vi "Configure Parametric Waveform.vi"(0 "VISA resource name":refnum<visa-resource-name>, 1 "Param. Wave Name":string, 2 "Prbs Parameters":cluster{"Prbs Type":u16, "Prbs Length [N]":i32}={"Prbs Type"=0, "Prbs Length [N]"=600} {"Prbs Type" items=[" PRBS-7", " PRBS-9", " PRBS-11", " PRBS-15", " PRBS-23", " PRBS-31"]}, 3 "Attribute":u16(ring) items=["Not Predefined", "Predefined"], 4 "Description":string, 5 "error in (no error)":errorcluster, 6 "Sampling Rate [Hz]":dbl=1200000000.0 format="%#_16g", 7 "Sine Parameters":T2={"Sine Cycles [N]"=1, "Sine Frequency [Hz]"=1000000.0, "Sine Phase [°]"=0, "Sine Length [N]"=600} {"Sine Frequency [Hz]" format="%#_16g"}, 8 "Sinc Parameters":T5={"Lobe Width [%]"=10.0, "Peak Position[%]"=50.0, "Sinc Length [N]"=600} {"Peak Position[%]" format="%#_16g"; "Lobe Width [%]" format="%#_16g"}, 9 "Exponential Parameters":T6={"Exponential Mode"=0, "Time Constant [s]"=5e-07, "Exp Length [N]"=600, "Exp Cycles [N]"=1} {"Time Constant [s]" format="%#_16g"; "Exponential Mode" items=["Rise", "Decay"]}, 10 "Auto Calc Option":u16(ring) items=["Length", "Sampling Rate", "Cycles", "Length & Cycles"], 11 "Pulse Parameters":T3={"Pulse Duty Cycle [%]"=50.0, "Pulse Pulse Delay[s]"=0.0, "Pulse Fall Time [s]"=1e-09, "Pulse Rise Time [s]"=1e-09, "Pulse Frequency [Hz]"=1000000.0, "Pulse Cycles [N]"=1, "Pulse Length [N]"=600} {"Pulse Frequency [Hz]" format="%#_16g"; "Pulse Rise Time [s]" format="%#_16g"; "Pulse Fall Time [s]" format="%#_16g"; "Pulse Pulse Delay[s]" format="%#_16g"; "Pulse Duty Cycle [%]" format="%#_16g"}, 12 "Wrap Around State":bool=TRUE, 13 "Sweep Parameters":T4={"Sweep Mode"=0, "Stop Frequency[Hz]"=5000000.0, "Start Frequency[Hz]"=1000000.0, "Sweep Length [N]"=600} {"Start Frequency[Hz]" format="%#_16g"; "Stop Frequency[Hz]" format="%#_16g"; "Sweep Mode" items=["Linear", "Logarithmic"]}, 15 "Square Parameters":T7={"Square Pulse Delay[s]"=0.0, "Sqaure Fall Time [s]"=1e-09, "Square Rise Time [s]"=1e-09, "Square Length [N]"=600, "Square Cycles [N]"=1, "Square Frequency [Hz]"=1000000.0} {"Square Frequency [Hz]" format="%#_16g"; "Square Rise Time [s]" format="%#_16g"; "Sqaure Fall Time [s]" format="%#_16g"; "Square Pulse Delay[s]" format="%#_16e"}, 16 "Multitone Parameters":T8(array[cluster])=[{"Tone Amplitude  [V]"=1.0, "Tone Phase  [°]"=0.0, "Tone Frequency [Hz]"=1000000.0}] {"Tone Frequency [Hz]" format="%#_16g"; "Tone Phase  [°]" format="%#_16g"; "Tone Amplitude  [V]" format="%#_16g"}, 18 "Parametric Type":u16(ring) items=["Sine", "Pulse", "Sweep", "Sinc", "Exponential", "Prbs", "Square", "Multitone"]) -> (14 "VISA resource name out":refnum<visa-resource-name>, 19 "error out":errorcluster)   [LabVIEW 2020, in "Active Technologies AWG3000.lvlib"]
uses:
  Active Technologies AWG3000.lvlib
panel:
  in  "Parametric Type Tabs":T1(tab)
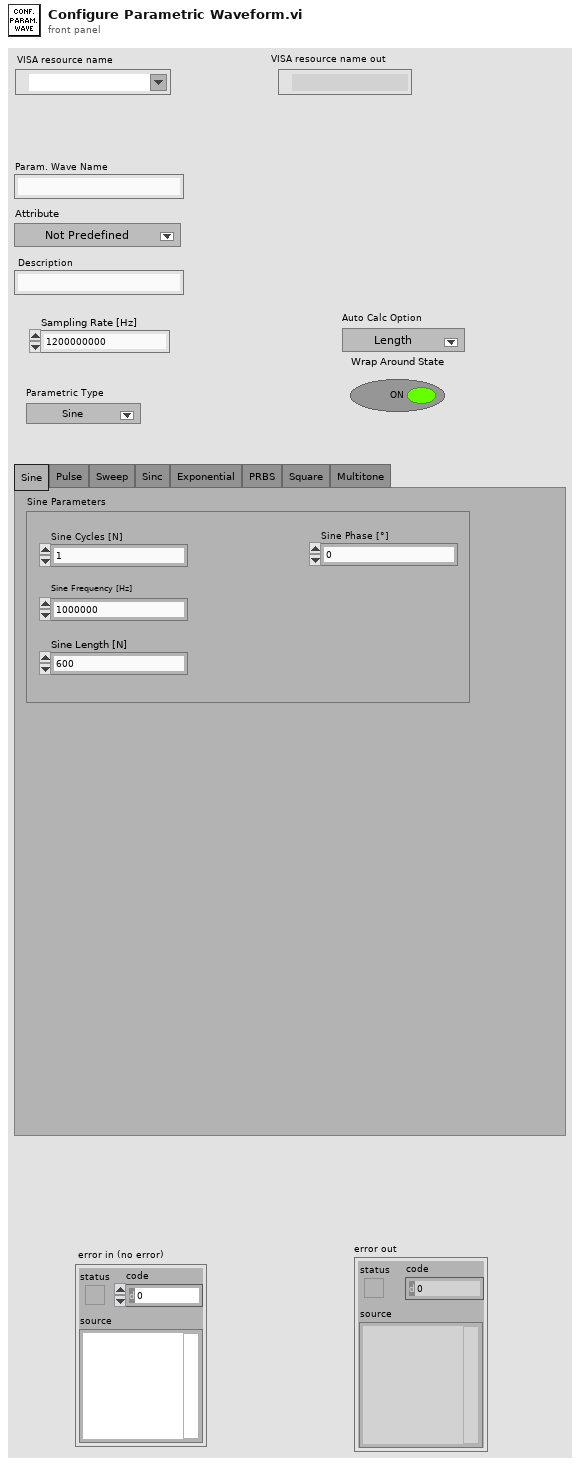
[diagram p1: front panel]
types:
  T1 = enum32{"Sine", "Pulse", "Sweep", "Sinc", "Exponential", "PRBS", "Square", "Multitone"}
  T2 = cluster{"Sine Cycles [N]":u32, "Sine Frequency [Hz]":dbl, "Sine Phase [°]":u32, "Sine Length [N]":i32}
  T3 = cluster{"Pulse Duty Cycle [%]":dbl, "Pulse Pulse Delay[s]":dbl, "Pulse Fall Time [s]":dbl, "Pulse Rise Time [s]":dbl, "Pulse Frequency [Hz]":dbl, "Pulse Cycles [N]":u32, "Pulse Length [N]":i32}
  T4 = cluster{"Sweep Mode":u16, "Stop Frequency[Hz]":dbl, "Start Frequency[Hz]":dbl, "Sweep Length [N]":i32}
  T5 = cluster{"Lobe Width [%]":dbl, "Peak Position[%]":dbl, "Sinc Length [N]":i32}
  T6 = cluster{"Exponential Mode":u16, "Time Constant [s]":dbl, "Exp Length [N]":i32, "Exp Cycles [N]":u32}
  T7 = cluster{"Square Pulse Delay[s]":dbl, "Sqaure Fall Time [s]":dbl, "Square Rise Time [s]":dbl, "Square Length [N]":i32, "Square Cycles [N]":u32, "Square Frequency [Hz]":dbl}
  T8 = cluster{"Tone Amplitude  [V]":dbl, "Tone Phase  [°]":dbl, "Tone Frequency [Hz]":dbl}[]
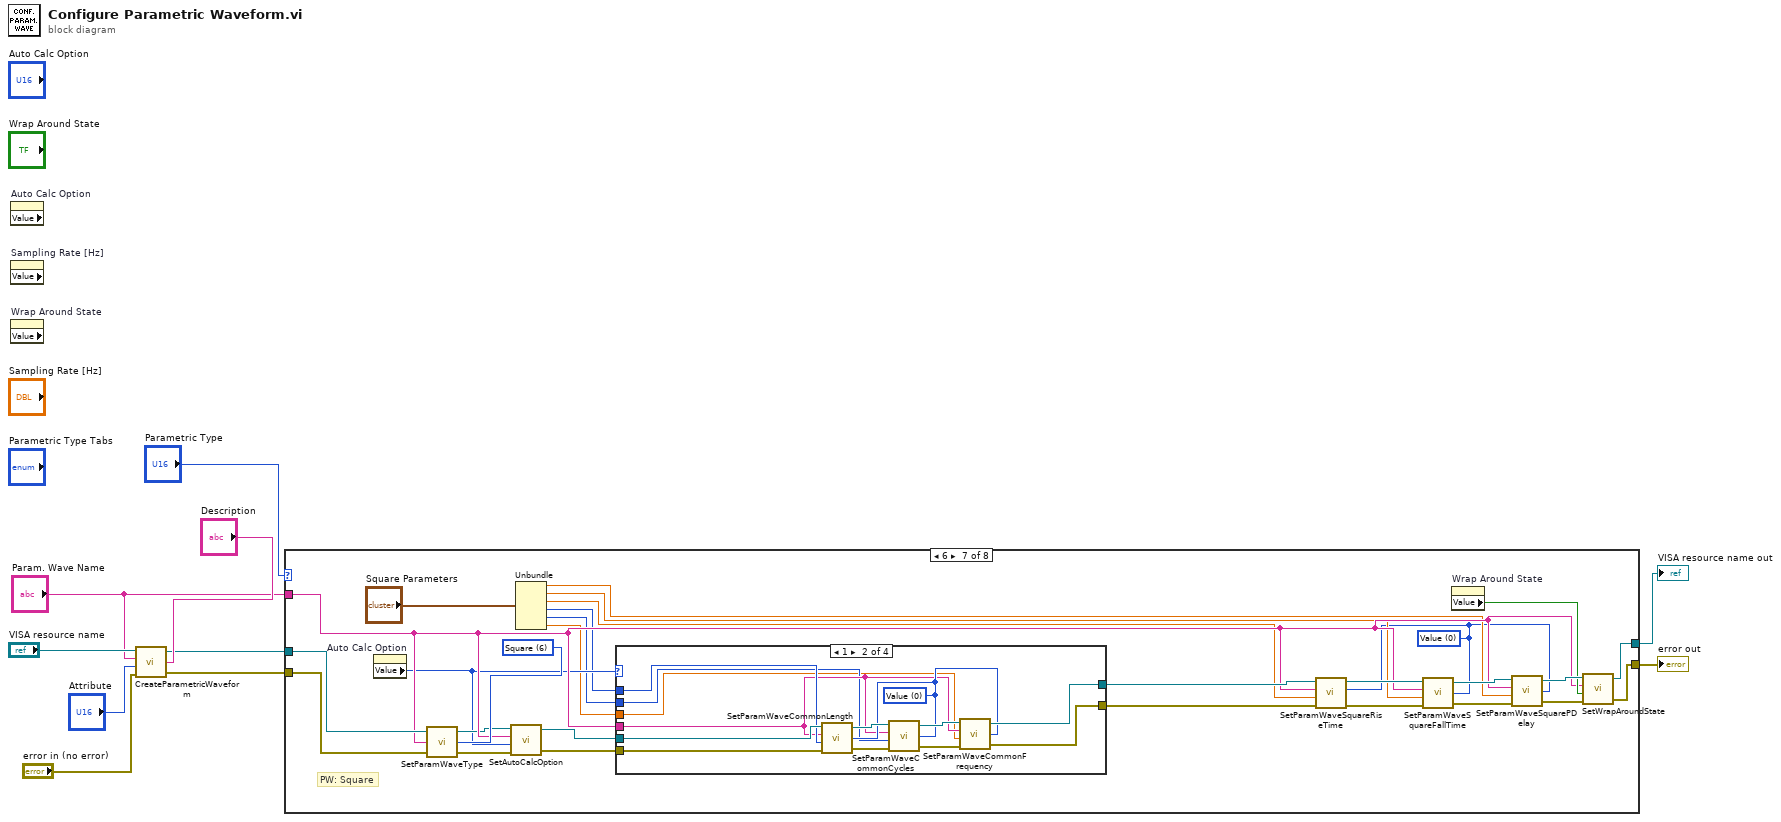
[diagram p0: block diagram]
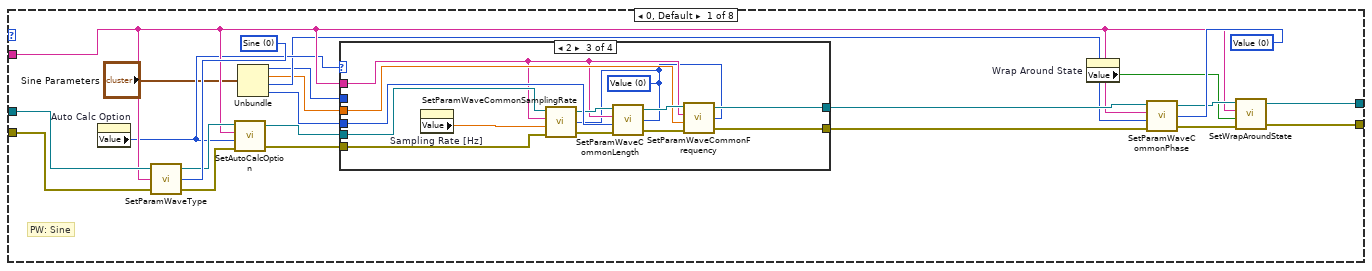
[diagram p2: hidden frame]
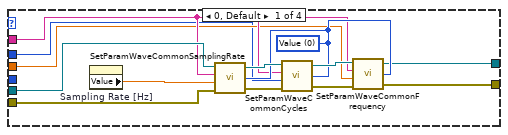
[diagram p3: hidden frame]
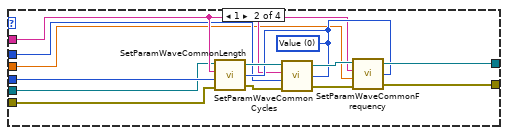
[diagram p4: hidden frame]
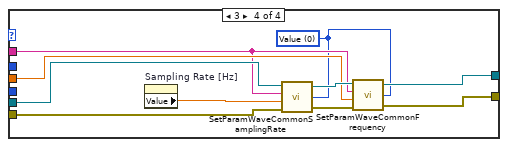
[diagram p5: hidden frame]
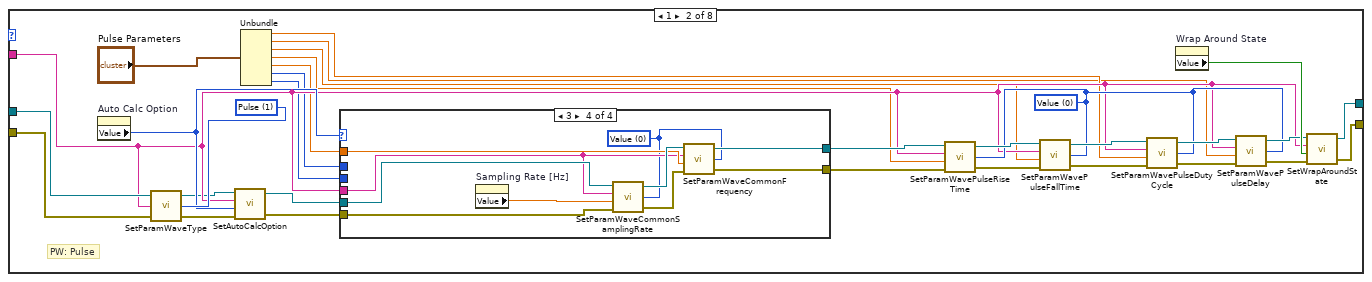
[diagram p6: hidden frame]
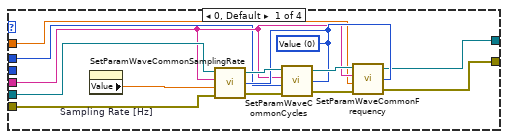
[diagram p7: hidden frame]
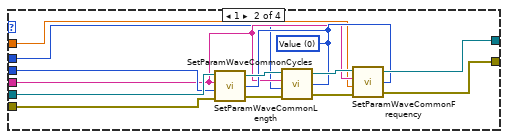
[diagram p8: hidden frame]
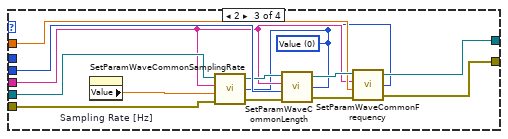
[diagram p9: hidden frame]
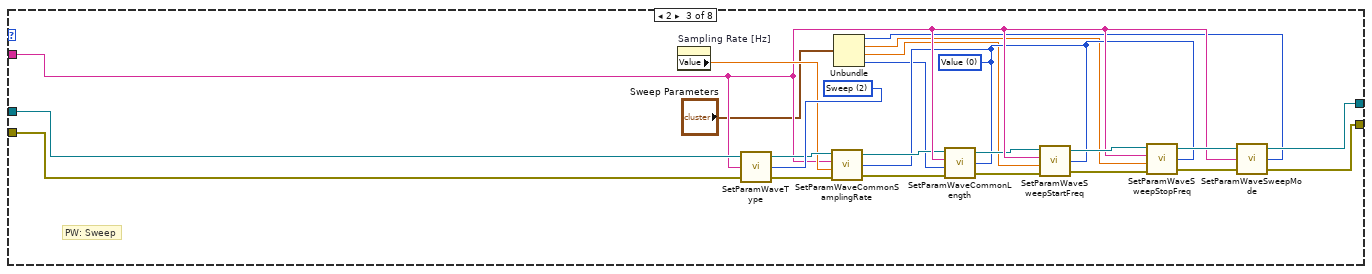
[diagram p10: hidden frame]
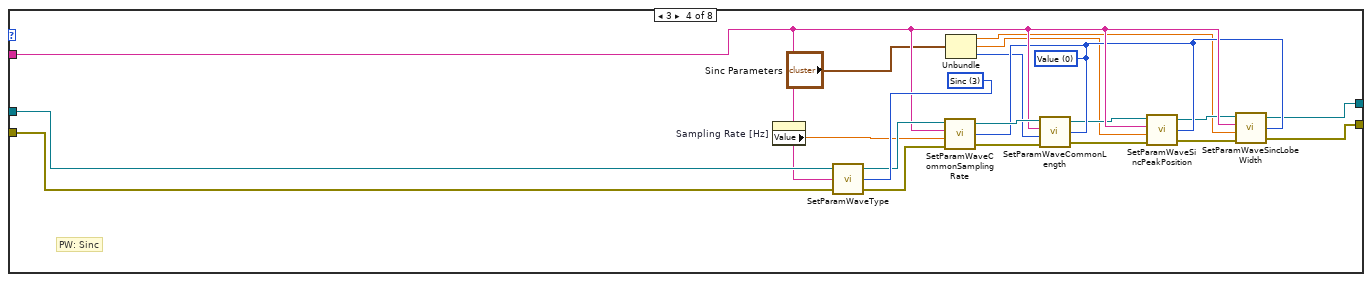
[diagram p11: hidden frame]
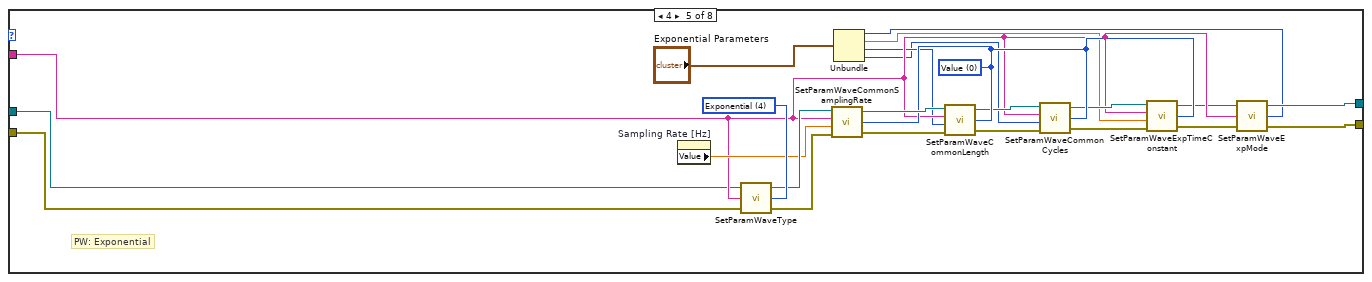
[diagram p12: hidden frame]
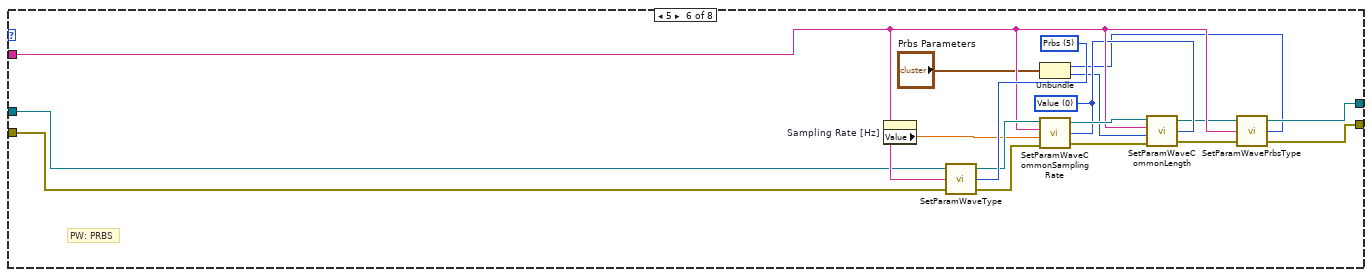
[diagram p13: hidden frame]
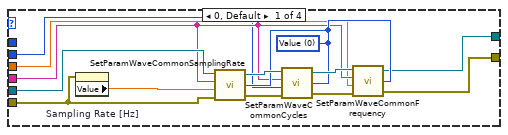
[diagram p14: hidden frame]
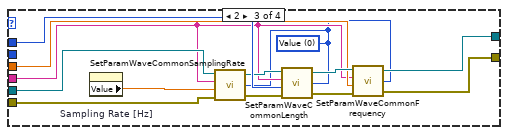
[diagram p15: hidden frame]
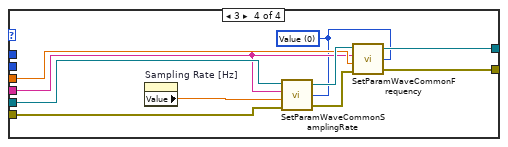
[diagram p16: hidden frame]
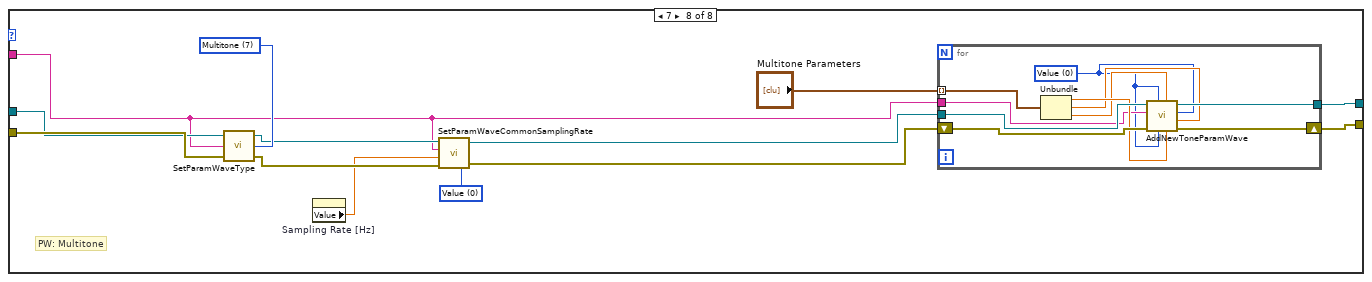
[diagram p17: hidden frame]
diagram:
  n1 = property on="Auto Calc Option" class="Ring (strict)" props=["Value"]() -> ()  [unwired: 2 in, 3 out]
  n2 = property on="Sampling Rate [Hz]" class="DigNum (strict)" props=["Value"]() -> ()  [unwired: 2 in, 3 out]
  n3 = property on="Wrap Around State" class="Bool (strict)" props=["Value"]() -> ()  [unwired: 2 in, 3 out]
  n4 = call "CreateParametricWaveform.vi"("Description"="Description", "error in (no error)"="error in (no error)", "Attribute"="Attribute", "Param. Wave Name"="Param. Wave Name", "VISA resource name"="VISA resource name") -> ("error out"=w4:errorcluster, "VISA resource name out"=w5:refnum<visa-resource-name>)
  n5 = case shown="6" "Parametric Type" {
    tunnel: "Param. Wave Name" -> [w19 w94 w172 w196 w217 w238 w258 w322]
    tunnel: w5 -> [w32 w110 w183 w198 w210 w237 w271 w333]
    tunnel: w4 -> [w31 w109 w182 w197 w211 w236 w270 w334]
    tunnel: [w23 w105 w181 w190 w213 w232 w266 w330] -> w2
    tunnel: [w22 w106 w180 w189 w212 w231 w265 w329] -> w3
    frame 0, Default {
      w27 = u16 0 items=["Value", "Default", "Minimum", "Maximum"] ("Selection")
      w30 = u16 0 items=["Sine", "Pulse", "Sweep", "Sinc", "Exponential", "Prbs", "Square", "Multitone"] ("ParamWaveType")
      # "PW: Sine"
      n6 = property on="Auto Calc Option" class="Ring (strict)"() -> ("Value"=w18:u16)  [unwired: 2 in, 2 out]
      n7 = call "SetParamWaveType.vi"("ParamWaveType"=w30, "error in (no error)"=w31, "ParamWave Name"=w19, "VISA resource name"=w32) -> ("error out"=w21:errorcluster, "VISA resource name out"=w20:refnum<visa-resource-name>)
      n8 = call "SetAutoCalcOption.vi"("error in (no error)"=w21, "Auto Calc Option"=w18, "ParamWave Name"=w19, "VISA resource name"=w20) -> ("error out"=w17:errorcluster, "VISA resource name out"=w16:refnum<visa-resource-name>)  [unwired: 1 in]
      n9 = Unbundle("Sine Parameters") -> ("Sine Cycles [N]"=w11:u32, "Sine Frequency [Hz]"=w13:dbl, "Sine Phase [°]"=w14:u32, "Sine Length [N]"=w12:i32)
      n10 = case shown="2" w18 {
        tunnel: w16 -> [w44 w46 w70 w81]
        tunnel: w17 -> [w43 w58 w69 w79]
        tunnel: w19 -> [w35 w50 w60 w75]
        tunnel: [w37 w52 w61 w73] -> w29
        tunnel: [w36 w53 w62 w74] -> w28
        tunnel: w13 -> [w34 w47 w63 w76]
        tunnel: w11 -> [w33 w49 _ _]
        tunnel: w12 -> [_ w57 w68 _]
        frame 0, Default {
          w38 = u16 0 items=["Value", "Default", "Minimum", "Maximum"] ("Selection")
          n11 = property on="Sampling Rate [Hz]" class="DigNum (strict)"() -> ("Value"=w45:dbl)  [unwired: 2 in, 2 out]
          n12 = call "SetParamWaveCommonSamplingRate.vi"("Selection"=w38, "error in (no error)"=w43, "Sampling Rate [Hz]"=w45, "ParamWave Name"=w35, "VISA resource name"=w44) -> ("error out"=w42:errorcluster, "VISA resource name out"=w41:refnum<visa-resource-name>)
          n13 = call "SetParamWaveCommonCycles.vi"("Selection"=w38, "error in (no error)"=w42, "Cycles [N]"=w33, "ParamWave Name"=w35, "VISA resource name"=w41) -> ("error out"=w39:errorcluster, "VISA resource name out"=w40:refnum<visa-resource-name>)
          n14 = call "SetParamWaveCommonFrequency.vi"("Selection"=w38, "error in (no error)"=w39, "Frequency [Hz]"=w34, "ParamWave Name"=w35, "VISA resource name"=w40) -> ("error out"=w37:errorcluster, "VISA resource name out"=w36:refnum<visa-resource-name>)
        }
        frame 1 {
          w51 = u16 0 items=["Value", "Default", "Minimum", "Maximum"] ("Selection")
          n15 = call "SetParamWaveCommonLength.vi"("Selection"=w51, "error in (no error)"=w58, "Length [N]"=w57, "ParamWave Name"=w50, "VISA resource name"=w46) -> ("error out"=w55:errorcluster, "VISA resource name out"=w56:refnum<visa-resource-name>)
          n16 = call "SetParamWaveCommonCycles.vi"("Selection"=w51, "error in (no error)"=w55, "Cycles [N]"=w49, "ParamWave Name"=w50, "VISA resource name"=w56) -> ("error out"=w48:errorcluster, "VISA resource name out"=w54:refnum<visa-resource-name>)
          n17 = call "SetParamWaveCommonFrequency.vi"("Selection"=w51, "error in (no error)"=w48, "Frequency [Hz]"=w47, "ParamWave Name"=w50, "VISA resource name"=w54) -> ("error out"=w52:errorcluster, "VISA resource name out"=w53:refnum<visa-resource-name>)
        }
        frame 2 {
          w59 = u16 0 items=["Value", "Default", "Minimum", "Maximum"] ("Selection")
          n18 = property on="Sampling Rate [Hz]" class="DigNum (strict)"() -> ("Value"=w71:dbl)  [unwired: 2 in, 2 out]
          n19 = call "SetParamWaveCommonSamplingRate.vi"("Selection"=w59, "error in (no error)"=w69, "Sampling Rate [Hz]"=w71, "ParamWave Name"=w60, "VISA resource name"=w70) -> ("error out"=w66:errorcluster, "VISA resource name out"=w67:refnum<visa-resource-name>)
          n20 = call "SetParamWaveCommonLength.vi"("Selection"=w59, "error in (no error)"=w66, "Length [N]"=w68, "ParamWave Name"=w60, "VISA resource name"=w67) -> ("error out"=w64:errorcluster, "VISA resource name out"=w65:refnum<visa-resource-name>)
          n21 = call "SetParamWaveCommonFrequency.vi"("Selection"=w59, "error in (no error)"=w64, "Frequency [Hz]"=w63, "ParamWave Name"=w60, "VISA resource name"=w65) -> ("error out"=w61:errorcluster, "VISA resource name out"=w62:refnum<visa-resource-name>)
        }
        frame 3 {
          w72 = u16 0 items=["Value", "Default", "Minimum", "Maximum"] ("Selection")
          n22 = property on="Sampling Rate [Hz]" class="DigNum (strict)"() -> ("Value"=w80:dbl)  [unwired: 2 in, 2 out]
          n23 = call "SetParamWaveCommonSamplingRate.vi"("Selection"=w72, "error in (no error)"=w79, "Sampling Rate [Hz]"=w80, "ParamWave Name"=w75, "VISA resource name"=w81) -> ("error out"=w77:errorcluster, "VISA resource name out"=w78:refnum<visa-resource-name>)
          n24 = call "SetParamWaveCommonFrequency.vi"("Selection"=w72, "error in (no error)"=w77, "Frequency [Hz]"=w76, "ParamWave Name"=w75, "VISA resource name"=w78) -> ("error out"=w73:errorcluster, "VISA resource name out"=w74:refnum<visa-resource-name>)
        }
      }
      n25 = property on="Wrap Around State" class="Bool (strict)"() -> ("Value"=w24:bool)  [unwired: 2 in, 2 out]
      n26 = call "SetParamWaveCommonPhase.vi"("Selection"=w27, "error in (no error)"=w29, "Phase [°]"=w14, "ParamWave Name"=w19, "VISA resource name"=w28) -> ("error out"=w25:errorcluster, "VISA resource name out"=w26:refnum<visa-resource-name>)
      n27 = call "SetWrapAroundState.vi"("error in (no error)"=w25, "Wrap Around State"=w24, "ParamWave Name"=w19, "VISA resource name"=w26) -> ("error out"=w22:errorcluster, "VISA resource name out"=w23:refnum<visa-resource-name>)  [unwired: 1 in]
    }
    frame 1 {
      w96 = u16 0 items=["Value", "Default", "Minimum", "Maximum"] ("Selection")
      w112 = u16 1 items=["Sine", "Pulse", "Sweep", "Sinc", "Exponential", "Prbs", "Square", "Multitone"] ("ParamWaveType")
      # "PW: Pulse"
      n28 = property on="Auto Calc Option" class="Ring (strict)"() -> ("Value"=w95:u16)  [unwired: 2 in, 2 out]
      n29 = call "SetParamWaveType.vi"("ParamWaveType"=w112, "error in (no error)"=w109, "ParamWave Name"=w94, "VISA resource name"=w110) -> ("error out"=w93:errorcluster, "VISA resource name out"=w92:refnum<visa-resource-name>)
      n30 = call "SetAutoCalcOption.vi"("error in (no error)"=w93, "Auto Calc Option"=w95, "ParamWave Name"=w94, "VISA resource name"=w92) -> ("error out"=w91:errorcluster, "VISA resource name out"=w90:refnum<visa-resource-name>)  [unwired: 1 in]
      n31 = Unbundle("Pulse Parameters") -> ("Pulse Duty Cycle [%]"=w88:dbl, "Pulse Pulse Delay[s]"=w87:dbl, "Pulse Fall Time [s]"=w86:dbl, "Pulse Rise Time [s]"=w85:dbl, "Pulse Frequency [Hz]"=w84:dbl, "Pulse Cycles [N]"=w83:u32, "Pulse Length [N]"=w82:i32)
      n32 = case shown="3" w95 {
        tunnel: w90 -> [w124 w138 w150 w161]
        tunnel: w91 -> [w123 w137 w149 w159]
        tunnel: w94 -> [w115 w129 w140 w155]
        tunnel: [w117 w131 w141 w153] -> w103
        tunnel: [w116 w132 w142 w154] -> w104
        tunnel: w84 -> [w114 w126 w143 w156]
        tunnel: w83 -> [w113 w128 _ _]
        tunnel: w82 -> [_ w136 w148 _]
        frame 0, Default {
          w118 = u16 0 items=["Value", "Default", "Minimum", "Maximum"] ("Selection")
          n33 = property on="Sampling Rate [Hz]" class="DigNum (strict)"() -> ("Value"=w125:dbl)  [unwired: 2 in, 2 out]
          n34 = call "SetParamWaveCommonSamplingRate.vi"("Selection"=w118, "error in (no error)"=w123, "Sampling Rate [Hz]"=w125, "ParamWave Name"=w115, "VISA resource name"=w124) -> ("error out"=w122:errorcluster, "VISA resource name out"=w121:refnum<visa-resource-name>)
          n35 = call "SetParamWaveCommonCycles.vi"("Selection"=w118, "error in (no error)"=w122, "Cycles [N]"=w113, "ParamWave Name"=w115, "VISA resource name"=w121) -> ("error out"=w119:errorcluster, "VISA resource name out"=w120:refnum<visa-resource-name>)
          n36 = call "SetParamWaveCommonFrequency.vi"("Selection"=w118, "error in (no error)"=w119, "Frequency [Hz]"=w114, "ParamWave Name"=w115, "VISA resource name"=w120) -> ("error out"=w117:errorcluster, "VISA resource name out"=w116:refnum<visa-resource-name>)
        }
        frame 1 {
          w130 = u16 0 items=["Value", "Default", "Minimum", "Maximum"] ("Selection")
          n37 = call "SetParamWaveCommonLength.vi"("Selection"=w130, "error in (no error)"=w137, "Length [N]"=w136, "ParamWave Name"=w129, "VISA resource name"=w138) -> ("error out"=w134:errorcluster, "VISA resource name out"=w135:refnum<visa-resource-name>)
          n38 = call "SetParamWaveCommonCycles.vi"("Selection"=w130, "error in (no error)"=w134, "Cycles [N]"=w128, "ParamWave Name"=w129, "VISA resource name"=w135) -> ("error out"=w127:errorcluster, "VISA resource name out"=w133:refnum<visa-resource-name>)
          n39 = call "SetParamWaveCommonFrequency.vi"("Selection"=w130, "error in (no error)"=w127, "Frequency [Hz]"=w126, "ParamWave Name"=w129, "VISA resource name"=w133) -> ("error out"=w131:errorcluster, "VISA resource name out"=w132:refnum<visa-resource-name>)
        }
        frame 2 {
          w139 = u16 0 items=["Value", "Default", "Minimum", "Maximum"] ("Selection")
          n40 = property on="Sampling Rate [Hz]" class="DigNum (strict)"() -> ("Value"=w151:dbl)  [unwired: 2 in, 2 out]
          n41 = call "SetParamWaveCommonSamplingRate.vi"("Selection"=w139, "error in (no error)"=w149, "Sampling Rate [Hz]"=w151, "ParamWave Name"=w140, "VISA resource name"=w150) -> ("error out"=w146:errorcluster, "VISA resource name out"=w147:refnum<visa-resource-name>)
          n42 = call "SetParamWaveCommonLength.vi"("Selection"=w139, "error in (no error)"=w146, "Length [N]"=w148, "ParamWave Name"=w140, "VISA resource name"=w147) -> ("error out"=w144:errorcluster, "VISA resource name out"=w145:refnum<visa-resource-name>)
          n43 = call "SetParamWaveCommonFrequency.vi"("Selection"=w139, "error in (no error)"=w144, "Frequency [Hz]"=w143, "ParamWave Name"=w140, "VISA resource name"=w145) -> ("error out"=w141:errorcluster, "VISA resource name out"=w142:refnum<visa-resource-name>)
        }
        frame 3 {
          w152 = u16 0 items=["Value", "Default", "Minimum", "Maximum"] ("Selection")
          n44 = property on="Sampling Rate [Hz]" class="DigNum (strict)"() -> ("Value"=w160:dbl)  [unwired: 2 in, 2 out]
          n45 = call "SetParamWaveCommonSamplingRate.vi"("Selection"=w152, "error in (no error)"=w159, "Sampling Rate [Hz]"=w160, "ParamWave Name"=w155, "VISA resource name"=w161) -> ("error out"=w157:errorcluster, "VISA resource name out"=w158:refnum<visa-resource-name>)
          n46 = call "SetParamWaveCommonFrequency.vi"("Selection"=w152, "error in (no error)"=w157, "Frequency [Hz]"=w156, "ParamWave Name"=w155, "VISA resource name"=w158) -> ("error out"=w153:errorcluster, "VISA resource name out"=w154:refnum<visa-resource-name>)
        }
      }
      n47 = call "SetParamWavePulseRiseTime.vi"("Selection"=w96, "error in (no error)"=w103, "Rise Time [s]"=w85, "ParamWave Name"=w94, "VISA resource name"=w104) -> ("error out"=w102:errorcluster, "VISA resource name out"=w101:refnum<visa-resource-name>)
      n48 = call "SetParamWavePulseFallTime.vi"("Selection"=w96, "error in (no error)"=w102, "Fall Time [s]"=w86, "ParamWave Name"=w94, "VISA resource name"=w101) -> ("error out"=w97:errorcluster, "VISA resource name out"=w100:refnum<visa-resource-name>)
      n49 = call "SetParamWavePulseDutyCycle.vi"("Selection"=w96, "error in (no error)"=w97, "Duty Cycle [%]"=w88, "ParamWave Name"=w94, "VISA resource name"=w100) -> ("error out"=w98:errorcluster, "VISA resource name out"=w99:refnum<visa-resource-name>)
      n50 = property on="Wrap Around State" class="Bool (strict)"() -> ("Value"=w111:bool)  [unwired: 2 in, 2 out]
      n51 = call "SetParamWavePulseDelay.vi"("Selection"=w96, "error in (no error)"=w98, "Pulse Delay[s]"=w87, "ParamWave Name"=w94, "VISA resource name"=w99) -> ("error out"=w107:errorcluster, "VISA resource name out"=w108:refnum<visa-resource-name>)
      n52 = call "SetWrapAroundState.vi"("error in (no error)"=w107, "Wrap Around State"=w111, "ParamWave Name"=w94, "VISA resource name"=w108) -> ("error out"=w106:errorcluster, "VISA resource name out"=w105:refnum<visa-resource-name>)  [unwired: 1 in]
    }
    frame 2 {
      w167 = u16 0 items=["Value", "Default", "Minimum", "Maximum"] ("Selection")
      w184 = u16 2 items=["Sine", "Pulse", "Sweep", "Sinc", "Exponential", "Prbs", "Square", "Multitone"] ("ParamWaveType")
      # "PW: Sweep"
      n53 = property on="Sampling Rate [Hz]" class="DigNum (strict)"() -> ("Value"=w175:dbl)  [unwired: 2 in, 2 out]
      n54 = call "SetParamWaveType.vi"("ParamWaveType"=w184, "error in (no error)"=w182, "ParamWave Name"=w172, "VISA resource name"=w183) -> ("error out"=w177:errorcluster, "VISA resource name out"=w176:refnum<visa-resource-name>)
      n55 = call "SetParamWaveCommonSamplingRate.vi"("Selection"=w167, "error in (no error)"=w177, "Sampling Rate [Hz]"=w175, "ParamWave Name"=w172, "VISA resource name"=w176) -> ("error out"=w170:errorcluster, "VISA resource name out"=w171:refnum<visa-resource-name>)
      n56 = Unbundle("Sweep Parameters") -> ("Sweep Mode"=w165:u16, "Stop Frequency[Hz]"=w164:dbl, "Start Frequency[Hz]"=w162:dbl, "Sweep Length [N]"=w163:i32)
      n57 = call "SetParamWaveCommonLength.vi"("Selection"=w167, "error in (no error)"=w170, "Length [N]"=w163, "ParamWave Name"=w172, "VISA resource name"=w171) -> ("error out"=w168:errorcluster, "VISA resource name out"=w169:refnum<visa-resource-name>)
      n58 = call "SetParamWaveSweepStartFreq.vi"("Selection"=w167, "error in (no error)"=w168, "Start Frequency[Hz]"=w162, "ParamWave Name"=w172, "VISA resource name"=w169) -> ("error out"=w178:errorcluster, "VISA resource name out"=w174:refnum<visa-resource-name>)
      n59 = call "SetParamWaveSweepStopFreq.vi"("Selection"=w167, "error in (no error)"=w178, "Stop Frequency[Hz]"=w164, "ParamWave Name"=w172, "VISA resource name"=w174) -> ("error out"=w179:errorcluster, "VISA resource name out"=w173:refnum<visa-resource-name>)
      n60 = call "SetParamWaveSweepMode.vi"("Sweep Mode"=w165, "error in (no error)"=w179, "ParamWave Name"=w172, "VISA resource name"=w173) -> ("error out"=w180:errorcluster, "VISA resource name out"=w181:refnum<visa-resource-name>)
    }
    frame 3 {
      w195 = u16 0 items=["Value", "Default", "Minimum", "Maximum"] ("Selection")
      w204 = u16 3 items=["Sine", "Pulse", "Sweep", "Sinc", "Exponential", "Prbs", "Square", "Multitone"] ("ParamWaveType")
      # "PW: Sinc"
      n61 = property on="Sampling Rate [Hz]" class="DigNum (strict)"() -> ("Value"=w201:dbl)  [unwired: 2 in, 2 out]
      n62 = call "SetParamWaveType.vi"("ParamWaveType"=w204, "error in (no error)"=w197, "ParamWave Name"=w196, "VISA resource name"=w198) -> ("error out"=w203:errorcluster, "VISA resource name out"=w202:refnum<visa-resource-name>)
      n63 = call "SetParamWaveCommonSamplingRate.vi"("Selection"=w195, "error in (no error)"=w203, "Sampling Rate [Hz]"=w201, "ParamWave Name"=w196, "VISA resource name"=w202) -> ("error out"=w199:errorcluster, "VISA resource name out"=w200:refnum<visa-resource-name>)
      n64 = Unbundle("Sinc Parameters") -> ("Lobe Width [%]"=w187:dbl, "Peak Position[%]"=w186:dbl, "Sinc Length [N]"=w185:i32)
      n65 = call "SetParamWaveCommonLength.vi"("Selection"=w195, "error in (no error)"=w199, "Length [N]"=w185, "ParamWave Name"=w196, "VISA resource name"=w200) -> ("error out"=w193:errorcluster, "VISA resource name out"=w194:refnum<visa-resource-name>)
      n66 = call "SetParamWaveSincPeakPosition.vi"("Selection"=w195, "error in (no error)"=w193, "Peak Position[%]"=w186, "ParamWave Name"=w196, "VISA resource name"=w194) -> ("error out"=w191:errorcluster, "VISA resource name out"=w192:refnum<visa-resource-name>)
      n67 = call "SetParamWaveSincLobeWidth.vi"("Selection"=w195, "error in (no error)"=w191, "Lobe Width [%]"=w187, "ParamWave Name"=w196, "VISA resource name"=w192) -> ("error out"=w189:errorcluster, "VISA resource name out"=w190:refnum<visa-resource-name>)
    }
    frame 4 {
      w221 = u16 0 items=["Value", "Default", "Minimum", "Maximum"] ("Selection")
      w227 = u16 4 items=["Sine", "Pulse", "Sweep", "Sinc", "Exponential", "Prbs", "Square", "Multitone"] ("ParamWaveType")
      # "PW: Exponential"
      n68 = property on="Sampling Rate [Hz]" class="DigNum (strict)"() -> ("Value"=w224:dbl)  [unwired: 2 in, 2 out]
      n69 = call "SetParamWaveType.vi"("ParamWaveType"=w227, "error in (no error)"=w211, "ParamWave Name"=w217, "VISA resource name"=w210) -> ("error out"=w226:errorcluster, "VISA resource name out"=w225:refnum<visa-resource-name>)
      n70 = call "SetParamWaveCommonSamplingRate.vi"("Selection"=w221, "error in (no error)"=w226, "Sampling Rate [Hz]"=w224, "ParamWave Name"=w217, "VISA resource name"=w225) -> ("error out"=w222:errorcluster, "VISA resource name out"=w223:refnum<visa-resource-name>)
      n71 = Unbundle("Exponential Parameters") -> ("Exponential Mode"=w208:u16, "Time Constant [s]"=w207:dbl, "Exp Length [N]"=w206:i32, "Exp Cycles [N]"=w205:u32)
      n72 = call "SetParamWaveCommonLength.vi"("Selection"=w221, "error in (no error)"=w222, "Length [N]"=w206, "ParamWave Name"=w217, "VISA resource name"=w223) -> ("error out"=w219:errorcluster, "VISA resource name out"=w220:refnum<visa-resource-name>)
      n73 = call "SetParamWaveCommonCycles.vi"("Selection"=w221, "error in (no error)"=w219, "Cycles [N]"=w205, "ParamWave Name"=w217, "VISA resource name"=w220) -> ("error out"=w216:errorcluster, "VISA resource name out"=w218:refnum<visa-resource-name>)
      n74 = call "SetParamWaveExpTimeConstant.vi"("Selection"=w221, "error in (no error)"=w216, "Time Constant [s]"=w207, "ParamWave Name"=w217, "VISA resource name"=w218) -> ("error out"=w214:errorcluster, "VISA resource name out"=w215:refnum<visa-resource-name>)
      n75 = call "SetParamWaveExpMode.vi"("Exponential Mode"=w208, "error in (no error)"=w214, "ParamWave Name"=w217, "VISA resource name"=w215) -> ("error out"=w212:errorcluster, "VISA resource name out"=w213:refnum<visa-resource-name>)
    }
    frame 5 {
      w235 = u16 0 items=["Value", "Default", "Minimum", "Maximum"] ("Selection")
      w244 = u16 5 items=["Sine", "Pulse", "Sweep", "Sinc", "Exponential", "Prbs", "Square", "Multitone"] ("ParamWaveType")
      # "PW: PRBS"
      n76 = property on="Sampling Rate [Hz]" class="DigNum (strict)"() -> ("Value"=w241:dbl)  [unwired: 2 in, 2 out]
      n77 = call "SetParamWaveType.vi"("ParamWaveType"=w244, "error in (no error)"=w236, "ParamWave Name"=w238, "VISA resource name"=w237) -> ("error out"=w243:errorcluster, "VISA resource name out"=w242:refnum<visa-resource-name>)
      n78 = Unbundle("Prbs Parameters") -> ("Prbs Type"=w229:u16, "Prbs Length [N]"=w228:i32)
      n79 = call "SetParamWaveCommonSamplingRate.vi"("Selection"=w235, "error in (no error)"=w243, "Sampling Rate [Hz]"=w241, "ParamWave Name"=w238, "VISA resource name"=w242) -> ("error out"=w239:errorcluster, "VISA resource name out"=w240:refnum<visa-resource-name>)
      n80 = call "SetParamWaveCommonLength.vi"("Selection"=w235, "error in (no error)"=w239, "Length [N]"=w228, "ParamWave Name"=w238, "VISA resource name"=w240) -> ("error out"=w233:errorcluster, "VISA resource name out"=w234:refnum<visa-resource-name>)
      n81 = call "SetParamWavePrbsType.vi"("Prbs Type"=w229, "error in (no error)"=w233, "ParamWave Name"=w238, "VISA resource name"=w234) -> ("error out"=w231:errorcluster, "VISA resource name out"=w232:refnum<visa-resource-name>)
    }
    frame 6 {
      w245 = u16 0 items=["Value", "Default", "Minimum", "Maximum"] ("Selection")
      w272 = u16 6 items=["Sine", "Pulse", "Sweep", "Sinc", "Exponential", "Prbs", "Square", "Multitone"] ("ParamWaveType")
      # "PW: Square"
      n82 = property on="Auto Calc Option" class="Ring (strict)"() -> ("Value"=w253:u16)  [unwired: 2 in, 2 out]
      n83 = call "SetParamWaveType.vi"("ParamWaveType"=w272, "error in (no error)"=w270, "ParamWave Name"=w258, "VISA resource name"=w271) -> ("error out"=w256:errorcluster, "VISA resource name out"=w257:refnum<visa-resource-name>)
      n84 = call "SetAutoCalcOption.vi"("error in (no error)"=w256, "Auto Calc Option"=w253, "ParamWave Name"=w258, "VISA resource name"=w257) -> ("error out"=w254:errorcluster, "VISA resource name out"=w255:refnum<visa-resource-name>)  [unwired: 1 in]
      n85 = Unbundle("Square Parameters") -> ("Square Pulse Delay[s]"=w246:dbl, "Sqaure Fall Time [s]"=w251:dbl, "Square Rise Time [s]"=w250:dbl, "Square Length [N]"=w247:i32, "Square Cycles [N]"=w248:u32, "Square Frequency [Hz]"=w249:dbl)
      n86 = case shown="1" w253 {
        tunnel: w255 -> [w285 w298 w311 w321]
        tunnel: w254 -> [w274 w297 w310 w320]
        tunnel: w258 -> [w277 w289 w301 w316]
        tunnel: [w279 w291 w302 w314] -> w263
        tunnel: [w278 w292 w303 w315] -> w264
        tunnel: w249 -> [w276 w286 w304 w317]
        tunnel: w248 -> [w275 w288 _ _]
        tunnel: w247 -> [_ w296 w309 _]
        frame 0, Default {
          w280 = u16 0 items=["Value", "Default", "Minimum", "Maximum"] ("Selection")
          n87 = property on="Sampling Rate [Hz]" class="DigNum (strict)"(error in=w274) -> ("Value"=w273:dbl)  [unwired: 1 in, 2 out]
          n88 = call "SetParamWaveCommonSamplingRate.vi"("Selection"=w280, "error in (no error)"=w274, "Sampling Rate [Hz]"=w273, "ParamWave Name"=w277, "VISA resource name"=w285) -> ("error out"=w284:errorcluster, "VISA resource name out"=w283:refnum<visa-resource-name>)
          n89 = call "SetParamWaveCommonCycles.vi"("Selection"=w280, "error in (no error)"=w284, "Cycles [N]"=w275, "ParamWave Name"=w277, "VISA resource name"=w283) -> ("error out"=w281:errorcluster, "VISA resource name out"=w282:refnum<visa-resource-name>)
          n90 = call "SetParamWaveCommonFrequency.vi"("Selection"=w280, "error in (no error)"=w281, "Frequency [Hz]"=w276, "ParamWave Name"=w277, "VISA resource name"=w282) -> ("error out"=w279:errorcluster, "VISA resource name out"=w278:refnum<visa-resource-name>)
        }
        frame 1 {
          w290 = u16 0 items=["Value", "Default", "Minimum", "Maximum"] ("Selection")
          n91 = call "SetParamWaveCommonLength.vi"("Selection"=w290, "error in (no error)"=w297, "Length [N]"=w296, "ParamWave Name"=w289, "VISA resource name"=w298) -> ("error out"=w294:errorcluster, "VISA resource name out"=w295:refnum<visa-resource-name>)
          n92 = call "SetParamWaveCommonCycles.vi"("Selection"=w290, "error in (no error)"=w294, "Cycles [N]"=w288, "ParamWave Name"=w289, "VISA resource name"=w295) -> ("error out"=w287:errorcluster, "VISA resource name out"=w293:refnum<visa-resource-name>)
          n93 = call "SetParamWaveCommonFrequency.vi"("Selection"=w290, "error in (no error)"=w287, "Frequency [Hz]"=w286, "ParamWave Name"=w289, "VISA resource name"=w293) -> ("error out"=w291:errorcluster, "VISA resource name out"=w292:refnum<visa-resource-name>)
        }
        frame 2 {
          w300 = u16 0 items=["Value", "Default", "Minimum", "Maximum"] ("Selection")
          n94 = property on="Sampling Rate [Hz]" class="DigNum (strict)"() -> ("Value"=w299:dbl)  [unwired: 2 in, 2 out]
          n95 = call "SetParamWaveCommonSamplingRate.vi"("Selection"=w300, "error in (no error)"=w310, "Sampling Rate [Hz]"=w299, "ParamWave Name"=w301, "VISA resource name"=w311) -> ("error out"=w307:errorcluster, "VISA resource name out"=w308:refnum<visa-resource-name>)
          n96 = call "SetParamWaveCommonLength.vi"("Selection"=w300, "error in (no error)"=w307, "Length [N]"=w309, "ParamWave Name"=w301, "VISA resource name"=w308) -> ("error out"=w305:errorcluster, "VISA resource name out"=w306:refnum<visa-resource-name>)
          n97 = call "SetParamWaveCommonFrequency.vi"("Selection"=w300, "error in (no error)"=w305, "Frequency [Hz]"=w304, "ParamWave Name"=w301, "VISA resource name"=w306) -> ("error out"=w302:errorcluster, "VISA resource name out"=w303:refnum<visa-resource-name>)
        }
        frame 3 {
          w313 = u16 0 items=["Value", "Default", "Minimum", "Maximum"] ("Selection")
          n98 = property on="Sampling Rate [Hz]" class="DigNum (strict)"() -> ("Value"=w312:dbl)  [unwired: 2 in, 2 out]
          n99 = call "SetParamWaveCommonSamplingRate.vi"("Selection"=w313, "error in (no error)"=w320, "Sampling Rate [Hz]"=w312, "ParamWave Name"=w316, "VISA resource name"=w321) -> ("error out"=w318:errorcluster, "VISA resource name out"=w319:refnum<visa-resource-name>)
          n100 = call "SetParamWaveCommonFrequency.vi"("Selection"=w313, "error in (no error)"=w318, "Frequency [Hz]"=w317, "ParamWave Name"=w316, "VISA resource name"=w319) -> ("error out"=w314:errorcluster, "VISA resource name out"=w315:refnum<visa-resource-name>)
        }
      }
      n101 = call "SetParamWaveSquareRiseTime.vi"("Selection"=w245, "error in (no error)"=w263, "Rise Time [s]"=w250, "ParamWave Name"=w258, "VISA resource name"=w264) -> ("error out"=w261:errorcluster, "VISA resource name out"=w262:refnum<visa-resource-name>)  [unwired: 1 in]
      n102 = call "SetParamWaveSquareFallTime.vi"("Selection"=w245, "error in (no error)"=w261, "Fall Time [s]"=w251, "ParamWave Name"=w258, "VISA resource name"=w262) -> ("error out"=w259:errorcluster, "VISA resource name out"=w260:refnum<visa-resource-name>)
      n103 = property on="Wrap Around State" class="Bool (strict)"() -> ("Value"=w267:bool)  [unwired: 2 in, 2 out]
      n104 = call "SetParamWaveSquarePDelay.vi"("Selection"=w245, "error in (no error)"=w259, "Pulse Delay[s]"=w246, "ParamWave Name"=w258, "VISA resource name"=w260) -> ("error out"=w269:errorcluster, "VISA resource name out"=w268:refnum<visa-resource-name>)
      n105 = call "SetWrapAroundState.vi"("error in (no error)"=w269, "Wrap Around State"=w267, "ParamWave Name"=w258, "VISA resource name"=w268) -> ("error out"=w265:errorcluster, "VISA resource name out"=w266:refnum<visa-resource-name>)  [unwired: 1 in]
    }
    frame 7 {
      w324 = u16 0 items=["Value", "Default", "Minimum", "Maximum"] ("Selection")
      w332 = u16 7 items=["Sine", "Pulse", "Sweep", "Sinc", "Exponential", "Prbs", "Square", "Multitone"] ("ParamWaveType")
      # "PW: Multitone"
      n106 = call "SetParamWaveType.vi"("ParamWaveType"=w332, "error in (no error)"=w334, "ParamWave Name"=w322, "VISA resource name"=w333) -> ("error out"=w327:errorcluster, "VISA resource name out"=w328:refnum<visa-resource-name>)
      n107 = property on="Sampling Rate [Hz]" class="DigNum (strict)"() -> ("Value"=w323:dbl)  [unwired: 2 in, 2 out]
      n108 = call "SetParamWaveCommonSamplingRate.vi"("Selection"=w324, "error in (no error)"=w327, "Sampling Rate [Hz]"=w323, "ParamWave Name"=w322, "VISA resource name"=w328) -> ("error out"=w325:errorcluster, "VISA resource name out"=w326:refnum<visa-resource-name>)
      n109 = for {
        tunnel: "Multitone Parameters" -> [w344] mode=indexing
        tunnel: w326 -> [w343]
        tunnel: [w341] -> w330
        shift-right: [w340] -> w329
        shift-left: w325 -> [w342]
        tunnel: w322 -> [w336]
        w335 = u16 0 items=["Value", "Default", "Minimum", "Maximum"] ("Amplitude Selection")
        n110 = Unbundle(w344) -> ("Tone Amplitude  [V]"=w339:dbl, "Tone Phase  [°]"=w338:dbl, "Tone Frequency [Hz]"=w337:dbl)
        n111 = call "AddNewToneParamWave.vi"("Phase  [°]"=w338, "Phase Selection"=w335, "Amplitude  [V]"=w339, "Frequency [Hz]"=w337, "Amplitude Selection"=w335, "Frequency Selection"=w335, "error in (no error)"=w342, "ParamWave Name"=w336, "VISA resource name"=w343) -> ("error out"=w340:errorcluster, "VISA resource name out"=w341:refnum<visa-resource-name>)  [unwired: 1 in]
      }
    }
  }
  "VISA resource name out" <- w2
  "error out" <- w3
